vi "Is Canceled.vi"(8 "error in (no error)":errorcluster, 11 "MeasurementContext in":refnum<class "MeasurementContext.lvclass">) -> (0 "error out":errorcluster, 2 "is canceled?":bool, 3 "MeasurementContext out":refnum<class "MeasurementContext.lvclass">)   [LabVIEW 2020, in "NI-DMM Measurement.lvlib" / "MeasurementContext.lvclass"]
uses:
  MeasurementContext.lvclass
  MeasurementContext.lvclass/MeasurementContext.ctl
  <vilib>/gRPC/LabVIEW gRPC Library/grpc-lvsupport-release.lvlib
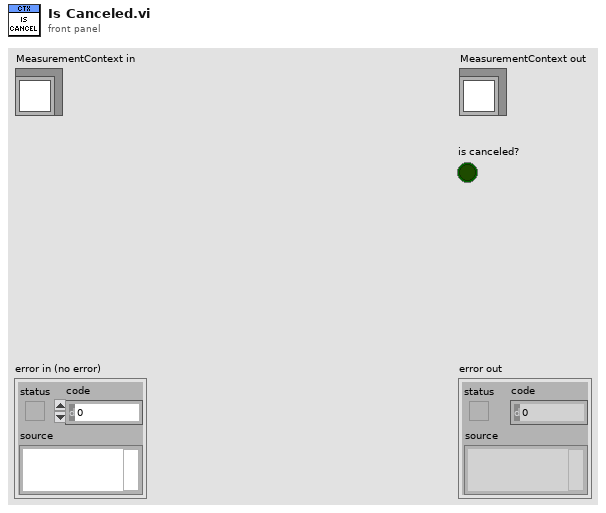
[diagram p1: front panel]
types:
  T1 = typedef "grpc-lvsupport-release.lvlib/grpcId.ctl" = u64
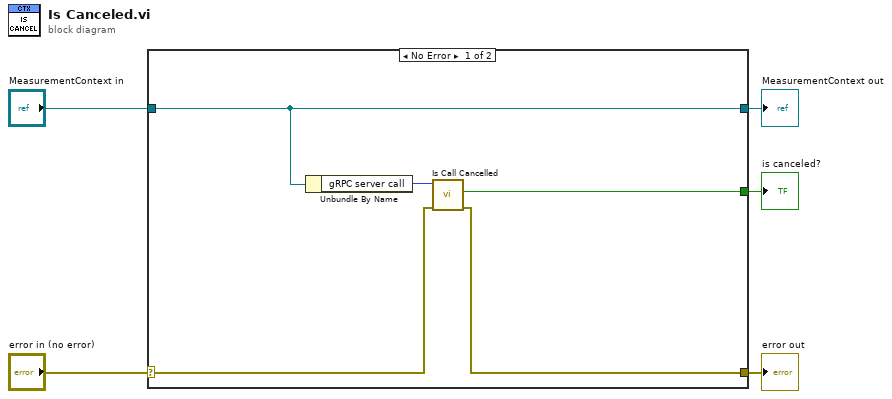
[diagram p0: block diagram]
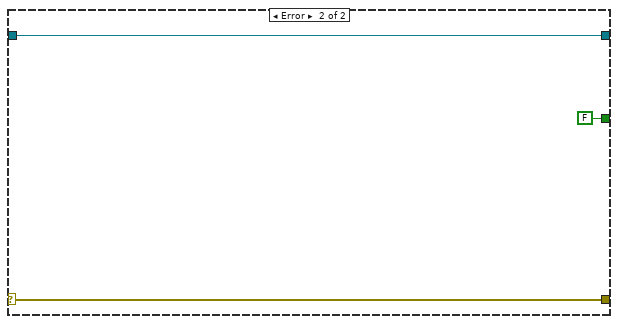
[diagram p2: hidden frame]
diagram:
  n1 = case shown="No Error" "error in (no error)" {
    selector: "error in (no error)" -> [w7 w13]
    tunnel: [w6 w13] -> w4
    tunnel: [w10 w12] -> w2
    tunnel: "MeasurementContext in" -> [w10 w12]
    tunnel: [w8 FALSE ("Is Cancelled")] -> w1
    frame No Error {
      n2 = Unbundle By Name(w10) -> ("gRPC server call"=w9:T1)
      n3 = call <vilib>:"Is Call Cancelled.vi"("error in"=w7, "gRPCid in"=w9) -> ("error out"=w6:errorcluster, "Is Cancelled"=w8:bool)  [unwired: 7 in, 1 out]
    }
    frame Error {
    }
  }
  "error out" <- w4
  "MeasurementContext out" <- w2
  "is canceled?" <- w1
